vi "Rebin Histogram with Dialog.vi"(8 "error in (no error)":errorcluster, 11 "Original Bin Histogram":cluster{"Axis":dbl[], "Histogram":dbl[]}) -> (0 "error out":errorcluster, 1 "OK?":bool, 3 "Rebinned Histogram":cluster{"Axis":dbl[], "Histogram":dbl[]})   [LabVIEW 2019, in "Histogram Window.lvlib"]
uses:
  Histogram Window.lvlib
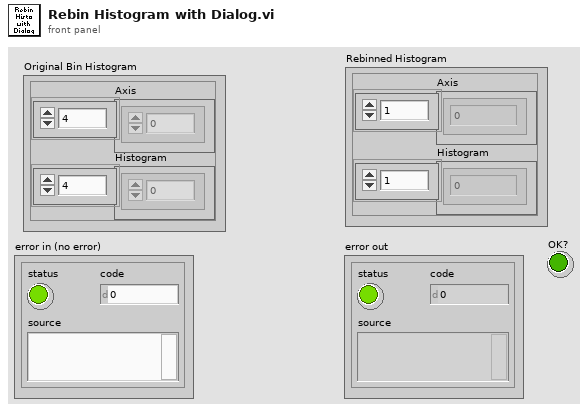
[diagram p1: front panel]
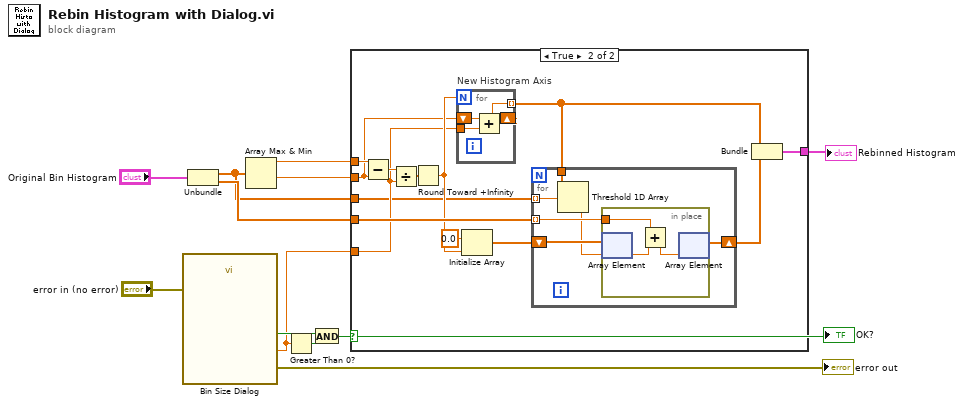
[diagram p0: block diagram]
diagram:
  n1 = call "Bin Size Dialog.vi"("error in (no error)"="error in (no error)") -> ("Bin Size"=w4:dbl, "OK"=w9:bool, "error out"=→"error out":errorcluster)  [unwired: 16 in]
  n2 = Unbundle("Original Bin Histogram") -> ("Axis"=w2:dbl[], "Histogram"=w3:dbl[])
  n3 = Array Max & Min(array=w2) -> (max value=w6:dbl, min value=w5:dbl)  [unwired: 2 out]
  n4 = Greater Than 0?(x=w4) -> (x > 0?=w10:bool)
  n5 = And(x=w9, y=w10) -> (x .and. y?=w8:bool)
  "OK?" <- w8
  n6 = case shown="True" w8 {
    tunnel: w6 -> [_ w25]
    tunnel: w5 -> [_ w18]
    tunnel: w4 -> [_ w17]
    tunnel: w3 -> [_ w21]
    tunnel: w2 -> [_ w16]
    tunnel: [_ w13] -> w1
    frame False {
    }
    frame True {
      n7 = Subtract(x=w25, y=w18) -> (x-y=w24:dbl)
      n8 = Divide(x=w24, y=w17) -> (x/y=w23:dbl)
      n9 = Round Toward +Infinity(x=w23) -> (ceil(x): smallest int >= x=w19:dbl)
      n10 = for "New Histogram Axis" {
        N: w19 -> [_]
        shift-right: [w27] -> _
        shift-left: w18 -> [w26]
        tunnel: w17 -> [w28]
        tunnel: [w26] -> w15 mode=indexing
        n11 = Add(x=w26, y=w28) -> (x+y=w27:dbl)
      }
      n12 = Initialize Array(0.0 ("element"), w19) -> (w20:dbl[])
      n13 = for {
        tunnel: w21 -> [w32] mode=indexing
        shift-right: [w33] -> w14
        shift-left: w20 -> [w34]
        tunnel: w16 -> [w30] mode=indexing
        tunnel: w15 -> [w31]
        n14 = Threshold 1D Array(2:w30, 3:w31) -> (0:w29:dbl)  [unwired: 1 in]
        n15 = in-place {
          in-place-border: w32 -> [w36]
          n16 = in-place-array #1(w34, w29) -> (w37:dbl)
          n17 = Add(x=w36, y=w37) -> (x+y=w35:dbl)
          n18 = in-place-array #1(w35) -> (w33:dbl[])  [unwired: 1 out]
        }
      }
      n19 = Bundle(w15, w14) -> (w13:cluster{dbl[], dbl[]})  [unwired: 1 in]
    }
  }
  "Rebinned Histogram" <- w1
